vi "_PC_Pub_FM openFile.vi"(7 "operation (0:open)":T1(ring), 8 "error in (no error)":errorcluster, 10 "openPath":path, 11 "FM in":refnum<class "FM.lvclass">) -> (0 "error out":errorcluster, 3 "FM out":refnum<class "FM.lvclass">)   [LabVIEW 2018, in "FM.lvclass"]
uses:
  FM.lvclass
  FM.lvclass/FM.ctl
  TDMSAdv.lvclass
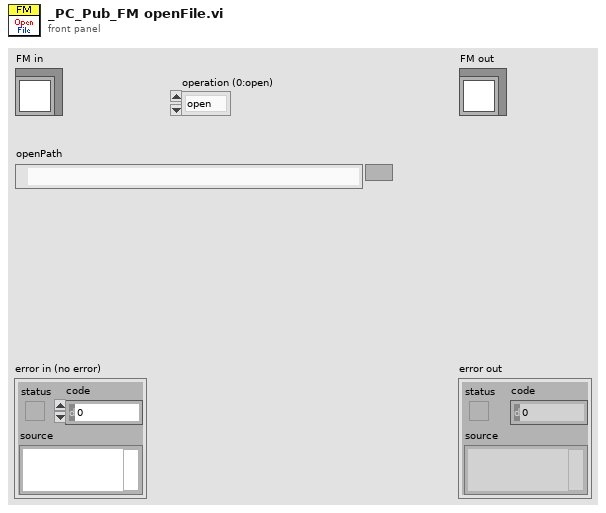
[diagram p1: front panel]
types:
  T1 = enum16{"open", "open or create", "create or replace", "create", "open (read-only)"}
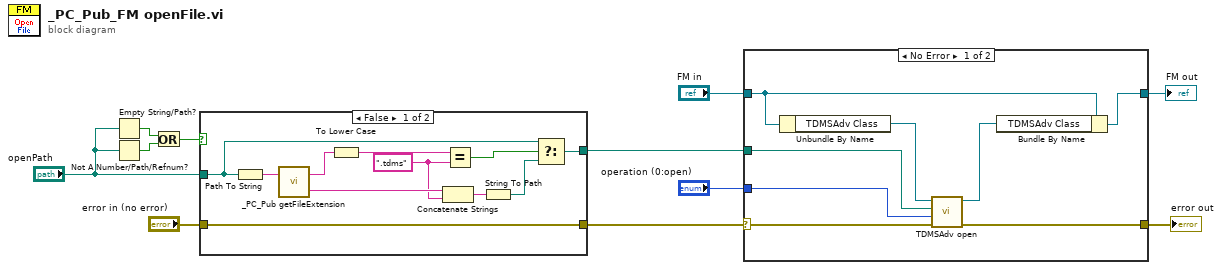
[diagram p0: block diagram]
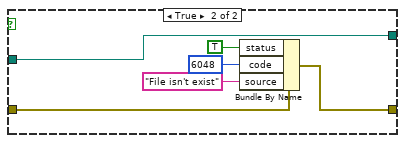
[diagram p3: hidden frame]
diagram:
  n1 = Empty String/Path?(string/path="openPath") -> (empty?=w11:bool)
  n2 = Not A Number/Path/Refnum?(number/path/refnum="openPath") -> (NaN/Path/Refnum?=w10:bool)
  n3 = Or(x=w11, y=w10) -> (x .or. y?=w9:bool)
  n4 = case shown="False" w9 {
    tunnel: "openPath" -> [w14 w28]
    tunnel: "error in (no error)" -> [w12 w27]
    tunnel: [w13 w28] -> w2
    tunnel: [w12 w23] -> w1
    frame False {
      w17 = ".tdms" ("x")
      n5 = Path To String(path=w14) -> (string=w22:string)
      n6 = call "_PC_Pub getFileExtension.vi"("Input"=w22) -> ("FileName"=w18:string, "ExtentionName"=w21:string)  [unwired: 1 in]
      n7 = To Lower Case(string=w21) -> (all lower case string=w20:string)
      n8 = Concatenate Strings(w18, w17) -> (w16:string)
      n9 = Equal?(x=w20, y=w17) -> (x = y?=w19:bool)
      n10 = String To Path(string=w16) -> (path=w15:path)
      n11 = Select(t=w14, s=w19, f=w15) -> (s? t:f=w13:path)
    }
    frame True {
      n12 = Bundle By Name(cluster=w27, "status"=TRUE, "code"=6048, "source"="File isn't exist") -> (w23:errorcluster)
    }
  }
  n13 = case shown="No Error" w1 {
    selector: w1 -> [w33 w38]
    tunnel: [w32 w38] -> w3
    tunnel: [w29 w37] -> w5
    tunnel: "FM in" -> [w31 w37]
    tunnel: w2 -> [w35 _]
    tunnel: "operation (0:open)" -> [w34 _]
    frame No Error {
      n14 = Unbundle By Name(w31) -> ("TDMSAdv Class"=w36:refnum<class "TDMSAdv.lvclass">)
      n15 = call "TDMSAdv open.vi"("error in (no error)"=w33, "operation (0:open)"=w34, "openPath"=w35, "TDMSAdv in"=w36) -> ("error out"=w32:errorcluster, "TDMSAdv out"=w30:refnum<class "TDMSAdv.lvclass">)  [unwired: 6 in]
      n16 = Bundle By Name(cluster=w31, "TDMSAdv Class"=w30) -> (w29:refnum<class "FM.lvclass">)
    }
    frame Error {
    }
  }
  "error out" <- w3
  "FM out" <- w5
